vi "LcWebView_PiePlot_Example.vi"() -> ()   [LabVIEW 2018, in "LcWebView.lvclass"]
doc: "Inject javascript arguments"
uses:
  LcWebView.lvclass
  plots/ctrls/PlotType.ctl
  plots/ctrls/PiePlotOption.ctl
  plots/ctrls/GenericPlotOption.ctl
  plots/ctrls/LegendPosition.ctl
  <userlib>/_OpenG.lib/numeric/numeric.llb/Random Number Within Range - DBL__ogtk.vi
  C:/Projects/LcWebView2/LcWebView/LcWebView_class/data/Microsoft.Web.WebView2.WinForms.dll
  data/Microsoft.Web.WebView2.WinForms.dll
panel:
  out "BrowserProcessId":u32
  out "Status Message":string
  in  "stop":bool
  in  "Web":refnum<k24>(container)
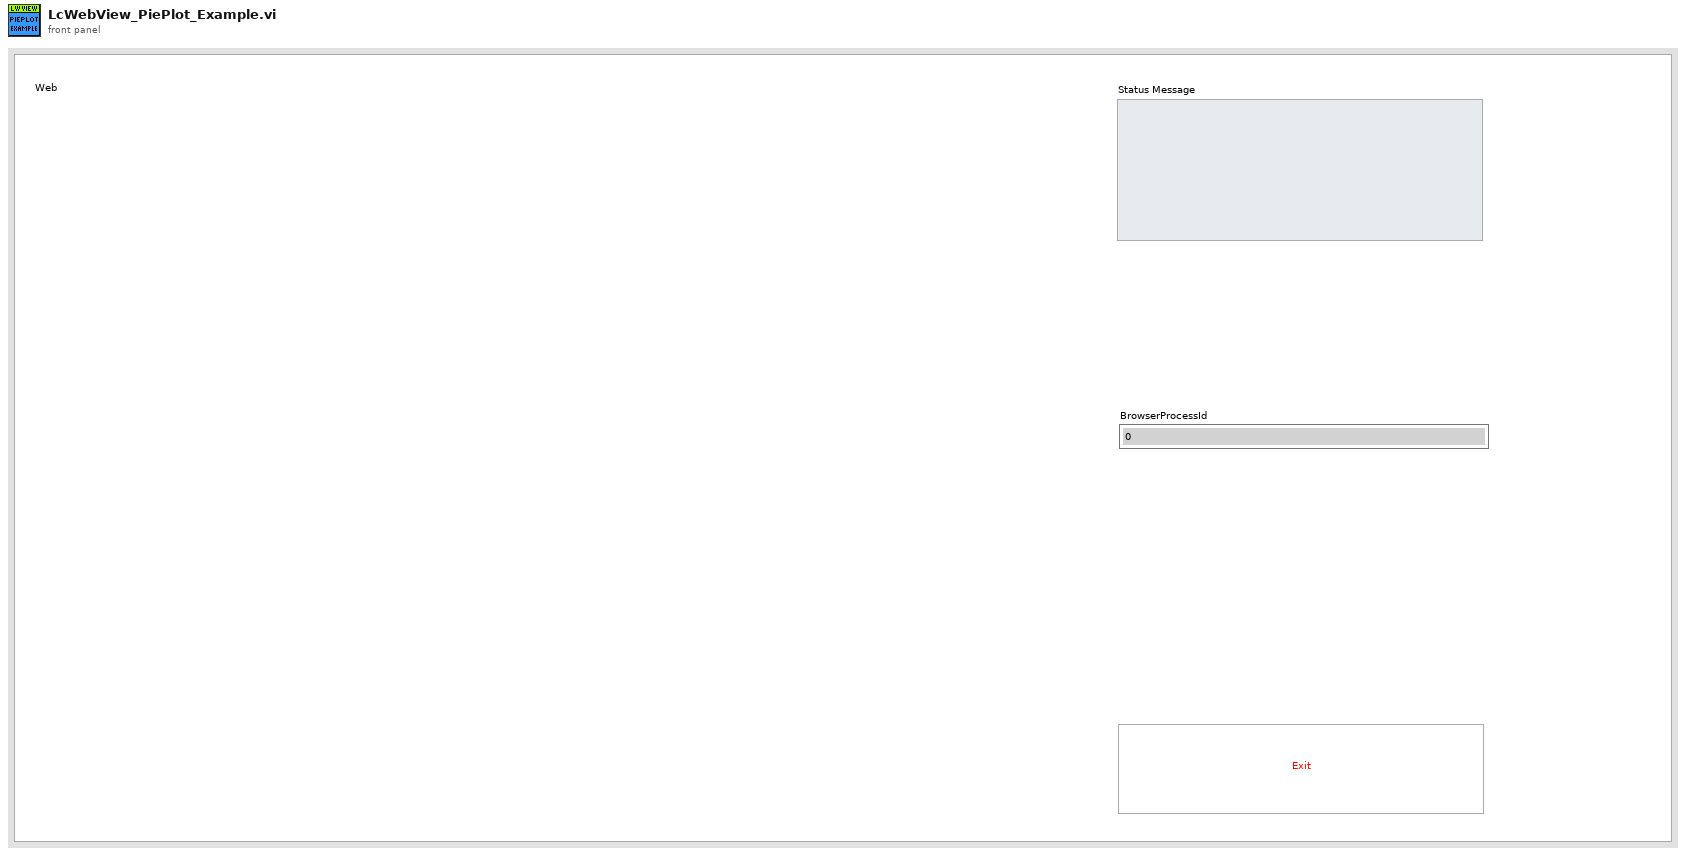
[diagram p1: front panel]
types:
  T1 = typedef "LcWebView.lvclass/GenericPlotOption.ctl" = cluster{"GraphTitle":string, "LegendDisplay":bool, "LegendPosition":T2}
  T2 = typedef "LcWebView.lvclass/LegendPosition.ctl" = enum16{"top", "right", "left", "bottom"}
  T3 = typedef "LcWebView.lvclass/PiePlotOption.ctl" = cluster{"cutoutPercentage":i32}
  T4 = typedef "LcWebView.lvclass/PlotType.ctl" = enum16{"bar", "line", "pie", "doughnut", "scatter", "radar", "bubble", "polarArea"}
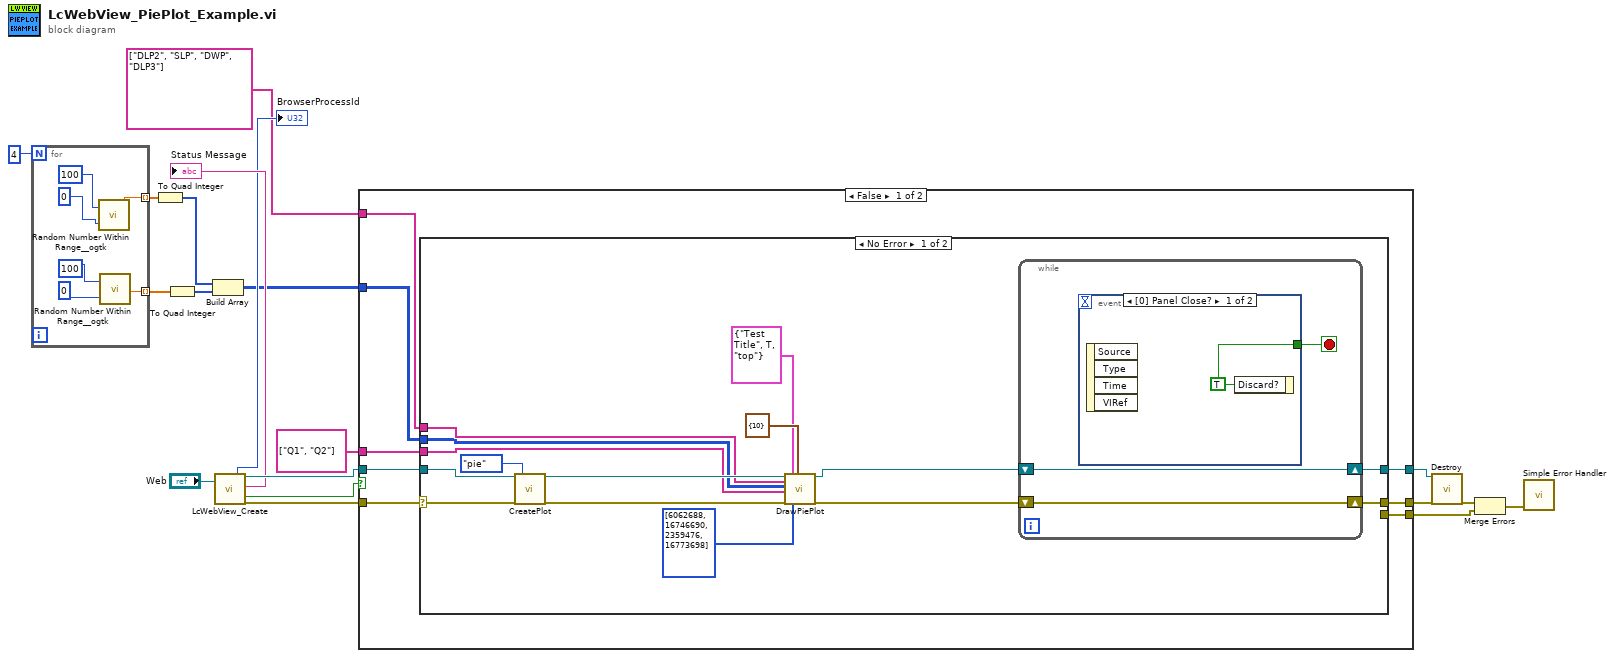
[diagram p0: block diagram]
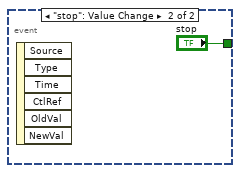
[diagram p2: hidden frame]
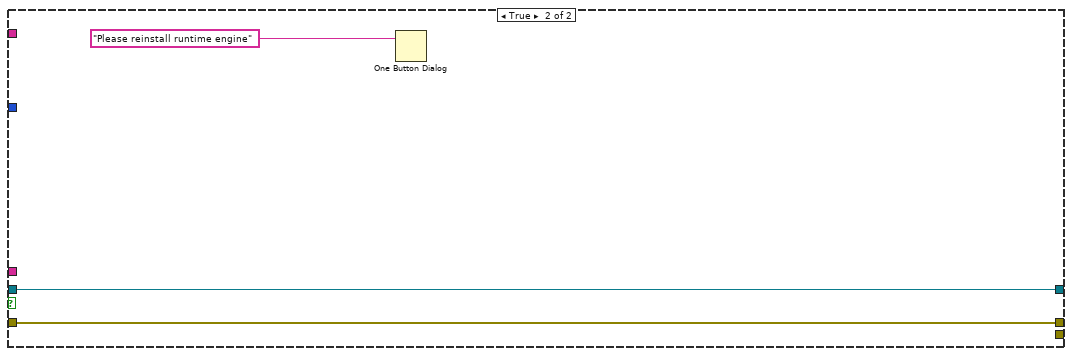
[diagram p4: hidden frame]
diagram:
  n1 = for {
    N: 4 -> [_]
    tunnel: [w23] -> w8 mode=indexing
    tunnel: [w20] -> w9 mode=indexing
    n2 = call-poly <userlib>:"Random Number Within Range__ogtk.vi"("High"=i64 100 ("upper bound (100)"), "Low"=i64 0 ("lower bound (-100)")) -> ("Random Number"=w23:dbl)  [unwired: 3 in]
    n3 = call-poly <userlib>:"Random Number Within Range__ogtk.vi"("High"=i64 100 ("upper bound (100)"), "Low"=i64 0 ("lower bound (-100)")) -> ("Random Number"=w20:dbl)  [unwired: 3 in]
  }
  n4 = To Quad Integer(1:w8) -> (0:w2:i64[])
  n5 = To Quad Integer(1:w9) -> (0:w1:i64[])
  n6 = Build Array(w2, w1) -> (w4:i64[][])
  n7 = call "LcWebView_Create.vi"("Webview container"="Web") -> ("BrowserProcessId"=→"BrowserProcessId":u32, "reference out"=w18:refnum<class "LcWebView.lvclass">, "Status Message"=→"Status Message":string, "Reinstall Runtime"=w11:bool, "Error Out"=w17:errorcluster)  [unwired: 11 in, 3 out]
  n8 = case shown="False" w11 {
    tunnel: w18 -> [w33 w58]
    tunnel: w17 -> [w32 w57]
    tunnel: [w31 w58] -> w16
    tunnel: [w29 w57] -> w15
    tunnel: [w30 _] -> w12
    tunnel: string[] ["DLP2", "SLP", "DWP", "DLP3"] ("DatasetLabels") -> [w28 _]
    tunnel: string[] ["Q1", "Q2"] ("PiePlot.PlotLabels") -> [w27 _]
    tunnel: w4 -> [w26 _]
    frame False {
      n9 = case shown="No Error" w32 {
        selector: w32 -> [w46 w54]
        tunnel: w33 -> [w47 w55]
        tunnel: [w42 w55] -> w31
        tunnel: [w48 _] -> w29
        tunnel: [_ w54] -> w30
        tunnel: w28 -> [w40 _]
        tunnel: w27 -> [w39 _]
        tunnel: w26 -> [w38 _]
        frame No Error {
          n10 = call-dynamic "CreatePlot.vi"("reference in"=w47, "Error In"=w46, "PlotType"=PlotType."pie") -> ("reference out"=w45:refnum<class "LcWebView.lvclass">, "Error Out"=w34:errorcluster)  [unwired: 15 in]
          n11 = call-dynamic "DrawPiePlot.vi"("reference in"=w45, "PiePlot.PlotLabels"=w40, "PiePlot.Dataset"=w38, "PiePlot.DatasetLabels"=w39, "Error In"=w34, "GenericPlotOptions"=T1 {"GraphTitle"="Test Title", "LegendDisplay"=TRUE, "LegendPosition"=enum."top"}, "PiePlot.PlotColours"=u32[] [6062688, 16746690, 2359476, 16773698] ("PlotColours"), "PiePlotOptions"=T3 {"cutoutPercentage"=10}) -> ("reference out"=w43:refnum<class "LcWebView.lvclass">, "Error Out"=w44:errorcluster)  [unwired: 10 in]
          n12 = while {
            shift-right: [w51] -> w42
            shift-left: w43 -> [w51]
            shift-right: [w50] -> w48
            shift-left: w44 -> [w50]
            stop <- w49 stop-if-true
            n13 = event shown="[0] Panel Close?" {
              selector: _ -> [_ _]
              dyn-events: _ -> [_ _]
              timeout: _ -> [_ _]
              tunnel: [w52 "stop"] -> w49
              event Panel Close? {
                w52 = TRUE ("Discard?")
                n14 = event-data() -> ()  [unwired: 1 in, 4 out]
                n15 = event-data("Discard?"=w52) -> ()  [unwired: 1 in, 1 out]
              }
              event "stop": Value Change {
                n16 = event-data() -> ()  [unwired: 1 in, 6 out]
              }
            }
          }
        }
        frame Error {
        }
      }
    }
    frame True {
      n17 = One Button Dialog(message="Please reinstall runtime engine") -> ()  [unwired: 1 in, 1 out]
    }
  }
  n18 = call-dynamic "Destroy.vi"("reference in"=w16, "Error In"=w15) -> ("Error Out"=w14:errorcluster)  [unwired: 16 in, 1 out]
  n19 = Merge Errors(w14, w12) -> (w3:errorcluster)
  n20 = call <vilib>:"Simple Error Handler.vi"("error in (no error)"=w3) -> ()  [unwired: 4 in, 5 out]
